vi "Calculate Particle Scores Ball.vi"(6 "Limit":dbl=80.0 format="%#_13g", 10 "Sorted Data":dbl[][](array[numeric])) -> (3 "Scores":T1[](array[typedef]))   [LabVIEW 2019]
doc: "Calculate scores based on the particle measurements. Calculated scores are for aspect ratio, area to convex hull area, and moment of inertia. These scores range between 0 and 100 and can be used to categorize particles as targets and non-targets."
uses:
  Vision Support Code/Target Fields.ctl
  <vilib>/Analysis/baseanly.llb/Mean (DBL).vi
  <vilib>/Analysis/NI_AALBase.lvlib
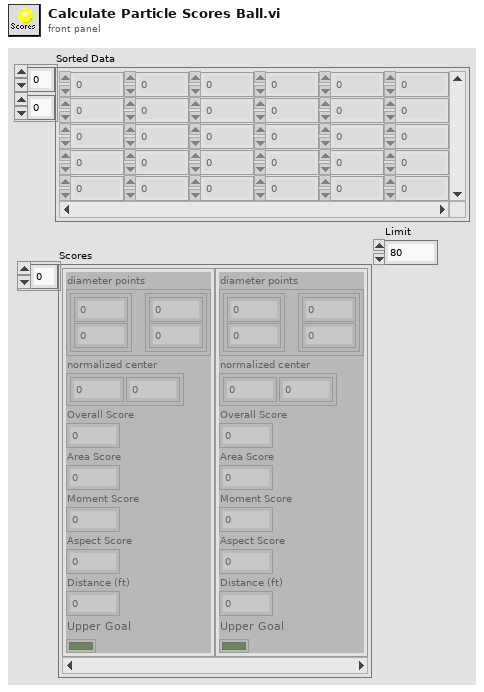
[diagram p1: front panel]
types:
  T1 = typedef "Target Fields.ctl" = cluster{"diameter points":cluster{"first point":cluster{"x":dbl, "y":dbl}, "projected point":cluster{"x":dbl, "y":dbl}}, "normalized center":cluster{"x":dbl, "y":dbl}, "Overall Score":dbl, "Area Score":dbl, "Moment Score":dbl, "Aspect Score":dbl, "Distance (ft)":dbl, "Upper Goal":bool}
  T2 = cluster{cluster{"Numeric":dbl, "Numeric":dbl}, cluster{"Numeric":dbl, "Numeric":dbl}}
  T3 = cluster{cluster{cluster{"Numeric":dbl, "Numeric":dbl}, cluster{"Numeric":dbl, "Numeric":dbl}}, "first point":cluster{"x":dbl, "y":dbl}, "mean":dbl, "Score":dbl, "Score":dbl, "Score":dbl, dbl, bool}
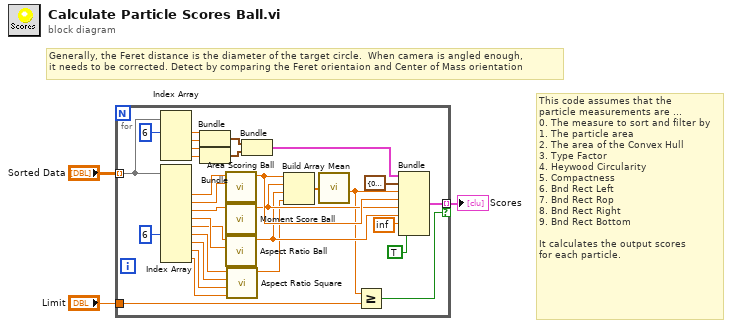
[diagram p0: block diagram]
diagram:
  # "Generally, the Feret distance is the diameter of the target circle.  When camera is angled enough,\nit needs to be corrected. Detect by comparing the Feret orientaion and Center of Mass orientation"
  # "This code assumes that the\nparticle measurements are ...\n0. The measure to sort and filter by\n1. The particle area\n2. The area of the Convex Hull\n3. Type Factor\n4. Heywood Circularity\n5. Compactness\n6. Bnd Rect Left\n7. Bnd Rect Rop\n8. Bnd Rect Right\n9. Bnd Rect Bottom\n\nIt calculates the output scores\nfor each particle."
  n1 = for {
    tunnel: "Sorted Data" -> [w30] mode=indexing
    tunnel: [w29] -> w2 mode=indexing if=w8
    tunnel: "Limit" -> [w18]
    n2 = Index Array(array=w30, index #1=6 ("index")) -> (element #1=w17:dbl, element #2=w16:dbl, element #3=w15:dbl, element #4=w14:dbl)  [unwired: 3 in]
    n3 = Index Array(array=w30, index #7=6 ("index")) -> (element #2=w26:dbl, element #3=w21:dbl, element #4=w23:dbl, element #5=w20:dbl, element #6=w19:dbl, element #7=w12:dbl, element #8=w11:dbl, element #9=w10:dbl, element #10=w9:dbl)  [unwired: 9 in, 1 out]
    n4 = Bundle("Numeric"=w17, "Numeric"=w16) -> (w28:cluster{"Numeric":dbl, "Numeric":dbl})  [unwired: 1 in]
    n5 = Bundle("Numeric"=w15, "Numeric"=w14) -> (w27:cluster{"Numeric":dbl, "Numeric":dbl})  [unwired: 1 in]
    n6 = call "Area Scoring Ball.vi"("Convex Hull Area"=w21, "Area"=w26) -> ("Score"=w25:dbl)  [unwired: 9 in]
    n7 = call "Moment Score Ball.vi"("Moment Factor"=w23) -> ("Score"=w24:dbl)  [unwired: 10 in]
    n8 = call "Aspect Ratio Ball.vi"("Circularity"=w20, "Compactness"=w19) -> ("Score"=w22:dbl)  [unwired: 9 in]
    n9 = call "Aspect Ratio Square.vi"("Bottom Left"=w9, "Top Left"=w10, "Bottom Right"=w11, "Top Right"=w12) -> ("Score"=w6:dbl)  [unwired: 7 in]
    n10 = Bundle(w28, w27) -> (w33:T2)  [unwired: 1 in]
    n11 = Build Array(w25, w24, w22, w6) -> (w5:dbl[])
    n12 = call-poly <vilib>:"Mean.vi"("X"=w5) -> ("mean"=w4:dbl)  [unwired: 1 out]
    n13 = Greater Or Equal?(x=w4, y=w18) -> (x >= y?=w8:bool)
    n14 = Bundle(w33, "first point"=cluster{"x":dbl, "y":dbl} {"x"=0.0, "y"=0.0}, "mean"=w4, "Score"=w25, "Score"=w24, "Score"=w22, inf, TRUE) -> (w29:T3)  [unwired: 1 in]
  }
  "Scores" <- w2
